vi "InsertData.vi"(8 "error in (no error)":errorcluster caption="错误输入（无错误）", 10 "检测电极":T1, 11 "table":string) -> (0 "error out":errorcluster caption="错误输出")   [LabVIEW 2014, in "DataBase.lvlib"]
uses:
  DataBase.lvlib
  <vilib>/addons/database/Connection.llb/DB Tools Open Connec (String).vi
  <vilib>/addons/database/NI_Database_API.lvlib
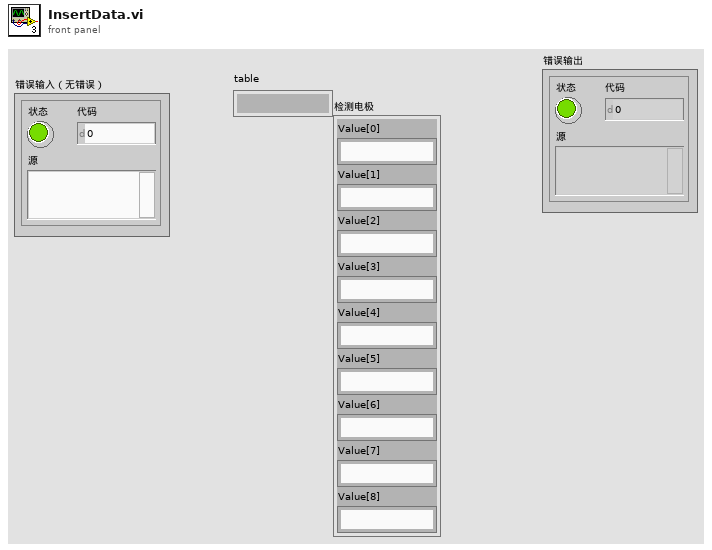
[diagram p1: front panel]
types:
  T1 = cluster{"Value[0]":string, "Value[1]":string, "Value[2]":string, "Value[3]":string, "Value[4]":string, "Value[5]":string, "Value[6]":string, "Value[7]":string, "Value[8]":string}
  T2 = typedef "NI_Database_API.lvlib/Conn ObjectReference.ctl" = refnum<k1>
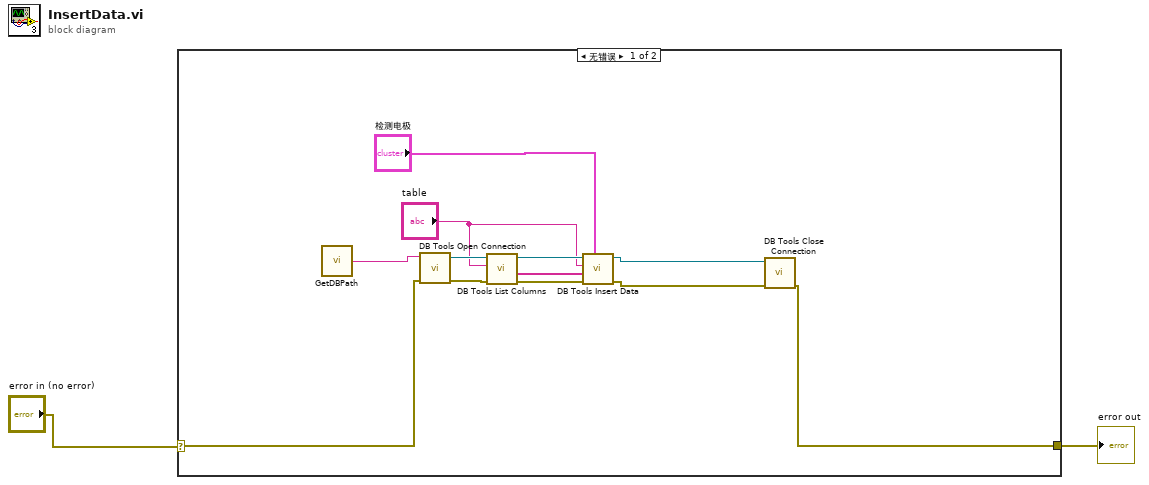
[diagram p0: block diagram]
diagram:
  n1 = case shown="无错误" "error in (no error)" {
    selector: "error in (no error)" -> [w11 w15]
    tunnel: [w8 w15] -> w1
    frame No Error {
      n2 = call "GetDBPath.vi"() -> ("Connection"=w14:string)  [unwired: 1 in]
      n3 = call-poly <vilib>:"DB Tools Open Connection.vi"("error in (no error)"=w11, "connection information"=w14) -> ("error out"=w10:errorcluster, "connection reference"=w13:T2)  [unwired: 6 in]
      n4 = call <vilib>:"DB Tools List Columns.vi"("error in (no error)"=w10, "table"="table", "connection reference"=w13) -> ("error out"=w9:errorcluster, "columns"=w5:string[], "connection reference out"=w12:T2)  [unwired: 1 in, 1 out]
      n5 = call <vilib>:"DB Tools Insert Data.vi"("data"="检测电极", "error in (no error)"=w9, "columns"=w5, "table"="table", "connection reference"=w12) -> ("error out"=w3:errorcluster, "connection reference out"=w4:T2)  [unwired: 5 in]
      n6 = call <vilib>:"DB Tools Close Connection.vi"("error in (no error)"=w3, "connection reference"=w4) -> ("error out"=w8:errorcluster)  [unwired: 5 in]
    }
    frame Error {
    }
  }
  "error out" <- w1
